vi "H2O Valve Control [B] (SubVI).vi"(0 "Water Valve Command":bool, 7 "ON PULSE":dbl=10.0, 11 "OFF PULSE":dbl=10.0) -> (4 "H2O Valve Signal":bool, 8 "Valve Active":bool, 15 "H2O Valve Reverse":bool)   [LabVIEW 2012]
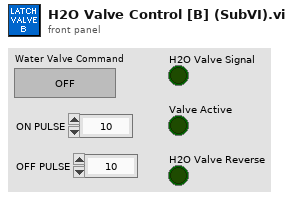
[diagram p1: front panel]
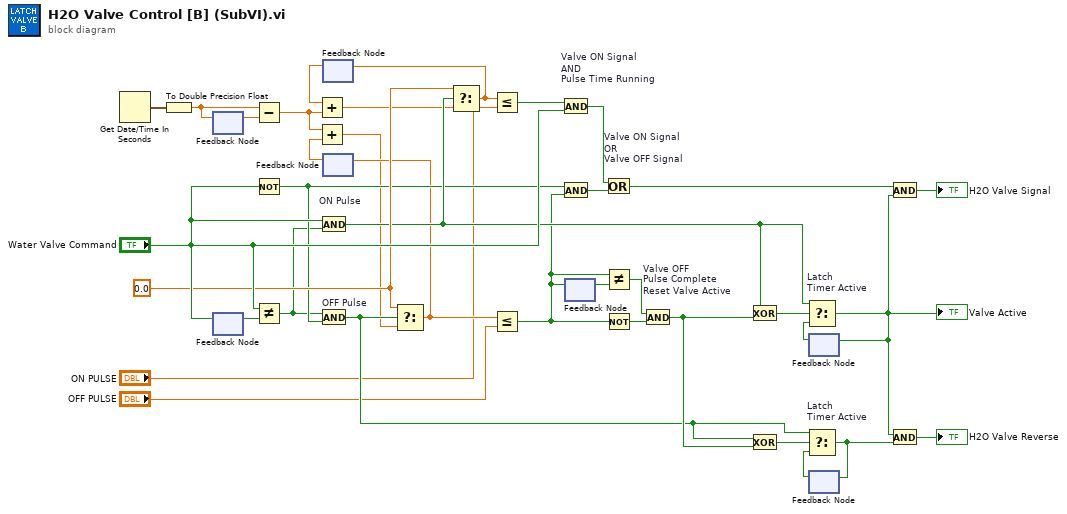
[diagram p0: block diagram]
diagram:
  w30 = 0.0 ("t")
  n1 = Get Date/Time In Seconds() -> (seconds since 1Jan1904=w6:timestamp)
  n2 = To Double Precision Float(number=w6) -> (double precision float=w7:dbl)
  n3 = feedback #1() -> (w5:dbl)  [unwired: 1 in]
  n4 = feedback-in #1(w7) -> ()
  n5 = feedback #2() -> (w1:bool)  [unwired: 1 in]
  n6 = feedback-in #2("Water Valve Command") -> ()
  n7 = Subtract(x=w7, y=w5) -> (x-y=w32:dbl)
  n8 = Not(x="Water Valve Command") -> (.not. x?=w13:bool)
  n9 = Not Equal?(x="Water Valve Command", y=w1) -> (x != y?=w2:bool)
  n10 = And "ON Pulse"(x="Water Valve Command", y=w2) -> (x .and. y?=w22:bool)
  n11 = And "OFF Pulse"(x=w2, y=w13) -> (x .and. y?=w25:bool)
  n12 = feedback #3() -> (w4:dbl)  [unwired: 1 in]
  n13 = Add(x=w4, y=w32) -> (x+y=w8:dbl)
  n14 = feedback #4() -> (w31:dbl)  [unwired: 1 in]
  n15 = Add(x=w32, y=w31) -> (x+y=w10:dbl)
  n16 = Select(t=w30, s=w25, f=w10) -> (s? t:f=w11:dbl)
  n17 = feedback-in #4(w11) -> ()
  n18 = Select(t=w30, s=w22, f=w8) -> (s? t:f=w9:dbl)
  n19 = feedback-in #3(w9) -> ()
  n20 = Less Or Equal?(x=w9, y="ON PULSE") -> (x <= y?=w36:bool)
  n21 = Less Or Equal?(x=w11, y="OFF PULSE") -> (x <= y?=w19:bool)
  n22 = And "Valve ON Signal\nAND\nPulse Time Running"(x=w36, y="Water Valve Command") -> (x .and. y?=w14:bool)
  n23 = And(x=w13, y=w19) -> (x .and. y?=w15:bool)
  n24 = feedback #5() -> (w17:bool)  [unwired: 1 in]
  n25 = feedback-in #5(w19) -> ()
  n26 = Or "Valve ON Signal\nOR\nValve OFF Signal"(x=w14, y=w15) -> (x .or. y?=w34:bool)
  n27 = Not Equal?(x=w19, y=w17) -> (x != y?=w18:bool)
  n28 = Not(x=w19) -> (.not. x?=w20:bool)
  n29 = And "Valve OFF\nPulse Complete\nReset Valve Active"(x=w18, y=w20) -> (x .and. y?=w26:bool)
  n30 = Exclusive Or(1:w26, 2:w22) -> (0:w16:bool)
  n31 = Exclusive Or(1:w26, 2:w25) -> (0:w23:bool)
  n32 = feedback #6() -> (w21:bool)  [unwired: 1 in]
  n33 = Select "Latch\nTimer Active"(t=w22, s=w16, f=w21) -> (s? t:f=w33:bool)
  "Valve Active" <- w33
  n34 = feedback-in #6(w33) -> ()
  n35 = feedback #7() -> (w24:bool)  [unwired: 1 in]
  n36 = Select "Latch\nTimer Active"(t=w25, s=w23, f=w24) -> (s? t:f=w28:bool)
  n37 = feedback-in #7(w28) -> ()
  n38 = And(x=w34, y=w33) -> (x .and. y?=→"H2O Valve Signal":bool)
  n39 = And(x=w33, y=w28) -> (x .and. y?=→"H2O Valve Reverse":bool)
